vi "Pnl Updts OFF.vi"(8 "error in":errorcluster) -> (0 "error out":errorcluster)   [LabVIEW 2023]
uses:
  <userlib>/_OpenG.lib/appcontrol/appcontrol.llb/openg_application_control.lvlib
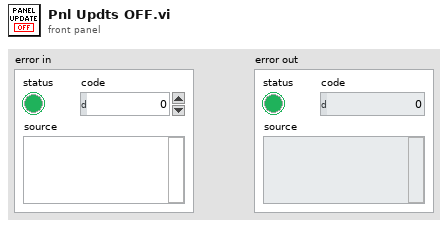
[diagram p1: front panel]
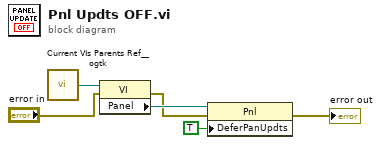
[diagram p0: block diagram]
diagram:
  n1 = call <userlib>:"Current VIs Parents Ref__ogtk.vi"() -> ("Calling VI's Reference"=w6:refnum<vi>)  [unwired: 2 in]
  n2 = property class="VI"(reference=w6, error in="error in") -> (error out=w3:errorcluster, "Panel"=w4:refnum<vi>)  [unwired: 1 out]
  n3 = property class="Pnl"(reference=w4, error in=w3, "DeferPanUpdts"=TRUE ("Defer Panel Updates")) -> (error out=→"error out":errorcluster)  [unwired: 1 out]
